vi "Get SMO Name.vi"(8 "error in (no error)":errorcluster, 11 "Instrument in":refnum<class "Instrument.lvclass">) -> (0 "error out":errorcluster, 2 "SMO Name":string, 3 "Instrument out":refnum<class "Instrument.lvclass">)   [LabVIEW 2019, in "Instrument.lvclass"]
uses:
  Instrument.lvclass
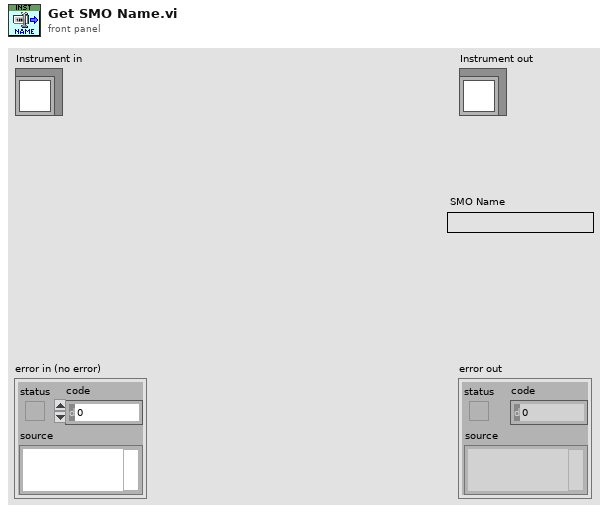
[diagram p1: front panel]
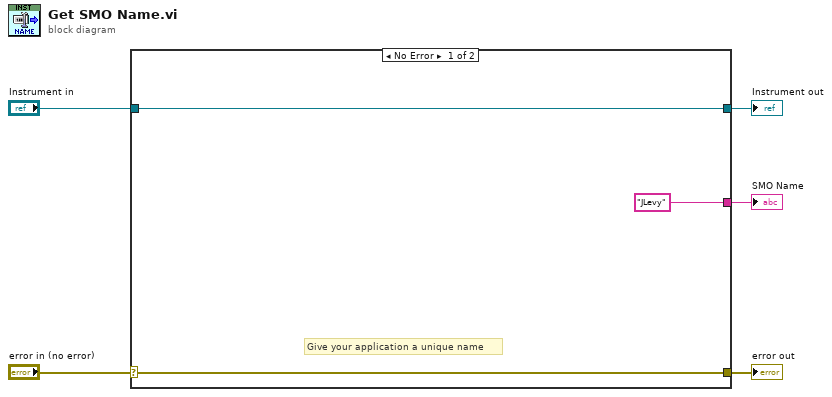
[diagram p0: block diagram]
diagram:
  n1 = case shown="No Error" "error in (no error)" {
    selector: "error in (no error)" -> [w7 w10]
    tunnel: [w7 w10] -> w4
    tunnel: [w8 w9] -> w2
    tunnel: "Instrument in" -> [w8 w9]
    tunnel: ["JLevy" ("SMO Name") _] -> w1
    frame No Error {
      # "Give your application a unique name"
    }
    frame Error {
    }
  }
  "error out" <- w4
  "Instrument out" <- w2
  "SMO Name" <- w1
